vi "Send InitDone.vi"(7 "Message Priority (Normal)":T2=enum."Normal", 8 "error in (no error)":errorcluster, 9 "instr error":errorcluster, 10 "Address":T1, 11 "Message Enqueuer":refnum<class "Message Enqueuer.lvclass">) -> (0 "error out":errorcluster, 3 "Message Enqueuer out":refnum<class "Message Enqueuer.lvclass">)   [LabVIEW 2023, in "InitDone Msg 2.lvclass"]
doc: "This VI sends the message to an actor."
uses:
  InitDone Msg 2.lvclass
  <vilib>/ActorFramework/Message Enqueuer/Message Enqueuer.lvclass
  <vilib>/ActorFramework/Message/Message.lvclass
  <vilib>/ActorFramework/Message Enqueuer/Message Priority.ctl
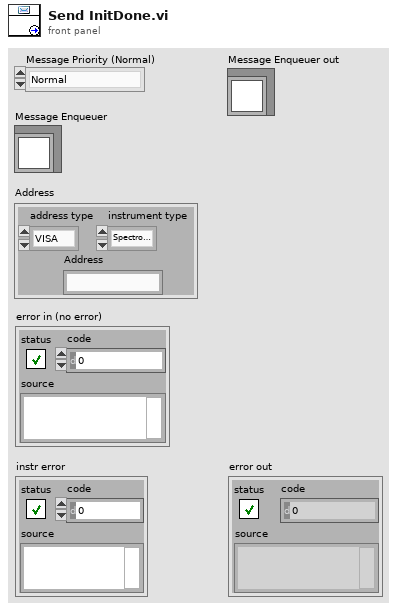
[diagram p1: front panel]
types:
  T1 = cluster{"address type":enum16{"VISA", "Index"}, "Address":string, "instrument type":enum16{"Spectrometer", "Camera", "Stepper"}}
  T2 = typedef "Actor Framework.lvlib/Message Enqueuer.lvclass/Message Priority.ctl" = enum16{"Low", "Normal", "High"}
  T3 = cluster{"Address":cluster{"address type":enum16{"VISA", "Index"}, "Address":string, "instrument type":enum16{"Spectrometer", "Camera", "Stepper"}}, "instr error":errorcluster}
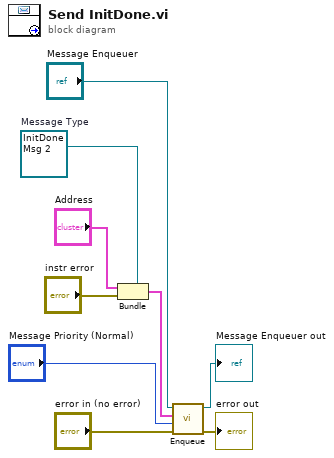
[diagram p0: block diagram]
diagram:
  w6 = refnum<class "InitDone Msg 2.lvclass"> refnum  # Message Type
  n1 = Bundle(cluster=w6, "Address"="Address", "instr error"="instr error") -> (w5:T3)
  n2 = call <vilib>:"Enqueue.vi"("error in (no error)"="error in (no error)", "Message Priority (Normal)"="Message Priority (Normal)", "Message"=w5, "Message Enqueuer in"="Message Enqueuer") -> ("error out"=→"error out":errorcluster, "Message Enqueuer out"=→"Message Enqueuer out":refnum<class "Message Enqueuer.lvclass">)  [unwired: 6 in]
